vi "Card Selector.vi"(9 "# Of Cards Total":i32, 10 "Card Array":bool[](array[boolean])) -> (2 "Card to use":i32)   [LabVIEW 2014, in "Universal Power Meter.lvlib" / "Universal Power Meter.lvclass"]
uses:
  Universal Power Meter.lvclass
panel:
  out "Numeric":i32
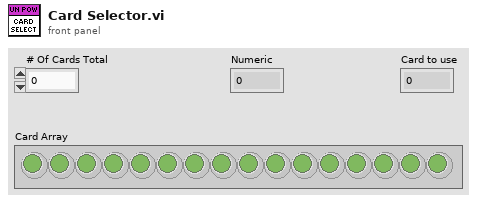
[diagram p1: front panel]
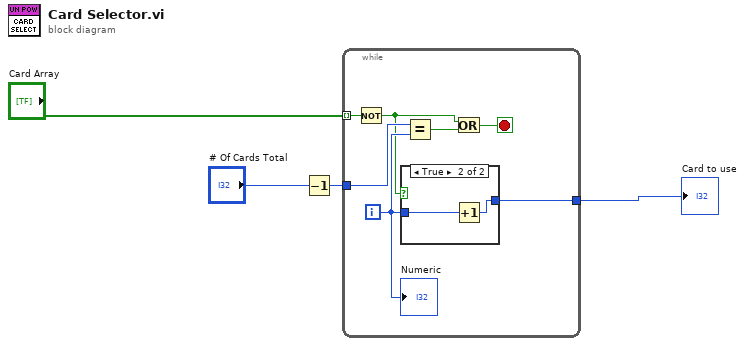
[diagram p0: block diagram]
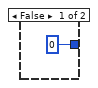
[diagram p2: hidden frame]
diagram:
  n1 = Decrement(x="# Of Cards Total") -> (x-1=w3:i32)
  n2 = while {
    tunnel: "Card Array" -> [w6] mode=indexing
    tunnel: w3 -> [w11]
    tunnel: [w9] -> w2
    i -> [w10]
    stop <- w7 stop-if-true
    n3 = Not(x=w6) -> (.not. x?=w5:bool)
    n4 = case shown="True" w5 {
      tunnel: w10 -> [_ w14]
      tunnel: [0 w13] -> w9
      frame False {
      }
      frame True {
        n5 = Increment(x=w14) -> (x+1=w13:i32)
      }
    }
    n6 = Equal?(x=w11, y=w10) -> (x = y?=w8:bool)
    n7 = Or(x=w5, y=w8) -> (x .or. y?=w7:bool)
    "Numeric" <- w10
  }
  "Card to use" <- w2
